vi "get position.vi"(8 "AI values":u32, 9 "DAC voltages":T1 {"pockels" max=4095 step=1; "y" max=4095 step=1; "x" max=4095 step=1}, 10 "useReadPosition":bool, 11 "tag lens trigger":bool) -> (0 "counts in last cycle":u16, 3 "current location":T2)   [LabVIEW 2010]
uses:
  common_typedefs/DAC_voltage_tagResonantr.ctl
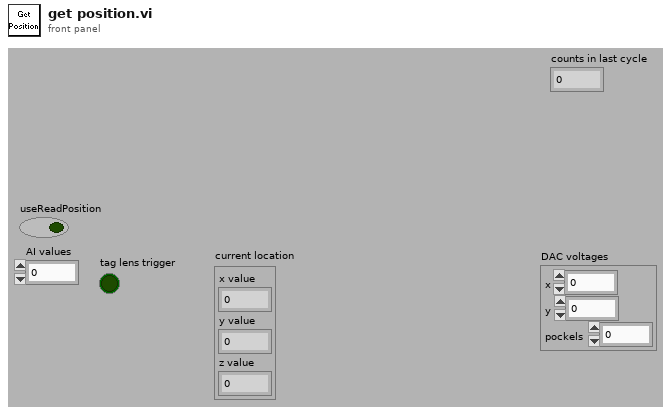
[diagram p1: front panel]
types:
  T1 = typedef "DAC_voltage_tagResonantr.ctl" = cluster{"x":i16, "y":i16, "pockels":i16}
  T2 = cluster{"x value":i16, "y value":i16, "z value":i16}
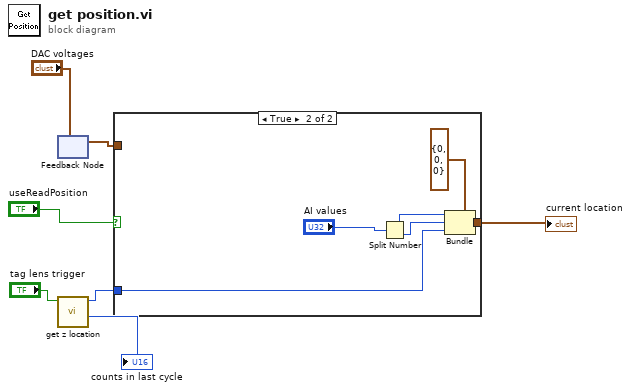
[diagram p0: block diagram]
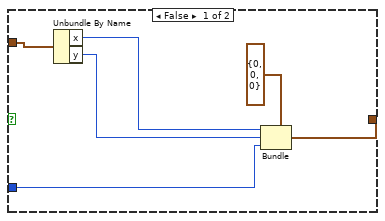
[diagram p2: hidden frame]
diagram:
  n1 = feedback-in #1("DAC voltages") -> ()
  n2 = feedback #1() -> (w3:T1)  [unwired: 1 in]
  n3 = call "get z location.vi"("tag lens trigger"="tag lens trigger") -> ("counts in last cycle"=→"counts in last cycle":u16, "z location"=w4:i16)  [unwired: 8 in, 1 out]
  n4 = case shown="True" "useReadPosition" {
    tunnel: [w11 w16] -> w2
    tunnel: w3 -> [w13 _]
    tunnel: w4 -> [w10 w15]
    frame False {
      n5 = Unbundle By Name(w13) -> ("x"=w9:i16, "y"=w8:i16)
      n6 = Bundle(cluster=T2 {"x value"=0, "y value"=0, "z value"=0} ("current location"), "x value"=w9, "y value"=w8, "z value"=w10) -> (w11:T2)
    }
    frame True {
      n7 = Split Number(x="AI values") -> (hi(x)=w18:u16, lo(x)=w17:u16)
      n8 = Bundle(cluster=T2 {"x value"=0, "y value"=0, "z value"=0} ("current location"), "x value"=w18, "y value"=w17, "z value"=w15) -> (w16:T2)
    }
  }
  "current location" <- w2
